vi "Globals.vi"() -> ()   [LabVIEW 2017, in "Server.lvlib"]
uses:
  Server.lvlib
  SubLibs/Oracle/OracleData.ctl
  SubLibs/Oracle/Oracle.lvlib
panel:
  in  "OracleData":T1
  in  "ErrorsToIgnore":i32[](array[numeric])
  out "TrackQueues?":bool
  in  "ClientTimeout (s)":u32
  in  "LogPath":path
  in  "MessageLogPath":path
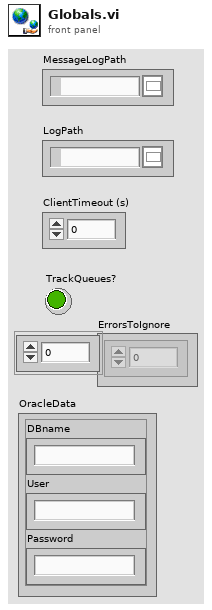
[diagram p1: front panel]
types:
  T1 = typedef "Server.lvlib/Oracle.lvlib/OracleData.ctl" = cluster{"DBname":string, "User":string, "Password":string}
diagram:
